vi "Method.vi"(4 "Value":refnum<class "Abs_Numeric.lvclass">) -> (1 "Result":refnum<class "ConvertTo_SGL.lvclass">)   [LabVIEW 2021, in "ConvertTo_SGL.lvclass"]
uses:
  ConvertTo_SGL.lvclass
  Abs_Types/Numeric/Abs_Numeric.lvclass
  ConvertTo_SGL.lvclass/ConvertTo_SGL.ctl
  Properties/Write Value.vi
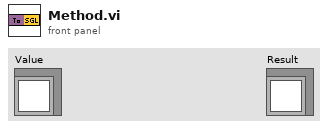
[diagram p1: front panel]
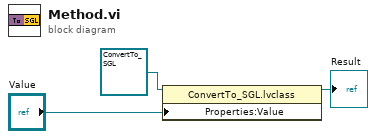
[diagram p0: block diagram]
diagram:
  n1 = property class="ConvertTo_SGL.lvclass"(reference=refnum<class "ConvertTo_SGL.lvclass"> refnum ("ConvertTo_DBL.lvclass"), "Properties:Value"="Value") -> (reference out=→"Result":refnum<class "ConvertTo_SGL.lvclass">)  [unwired: 1 in, 1 out]
